vi "StimFile-Create.vi"(0 "File":T1, 7 "Npts":i32=-1, 11 "error in (no error)":errorcluster) -> (4 "File out":T1, 8 "Y":dbl[](array[numeric]), 15 "error out":errorcluster)   [LabVIEW 2020]
uses:
  StimFile-Params.ctl
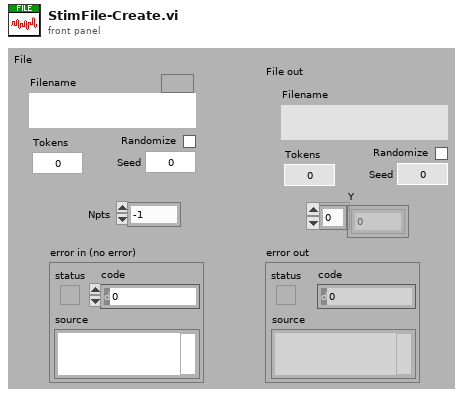
[diagram p1: front panel]
types:
  T1 = typedef "StimFile-Params.ctl" = cluster{"Filename":path, "Signal":dbl[], "Channel":i32, "stream":bool, "offset":i32, "nreps":i32, "loops":i32, "Randomize":bool, "order":i32[], "Seed":i32, "Tokens":i32}
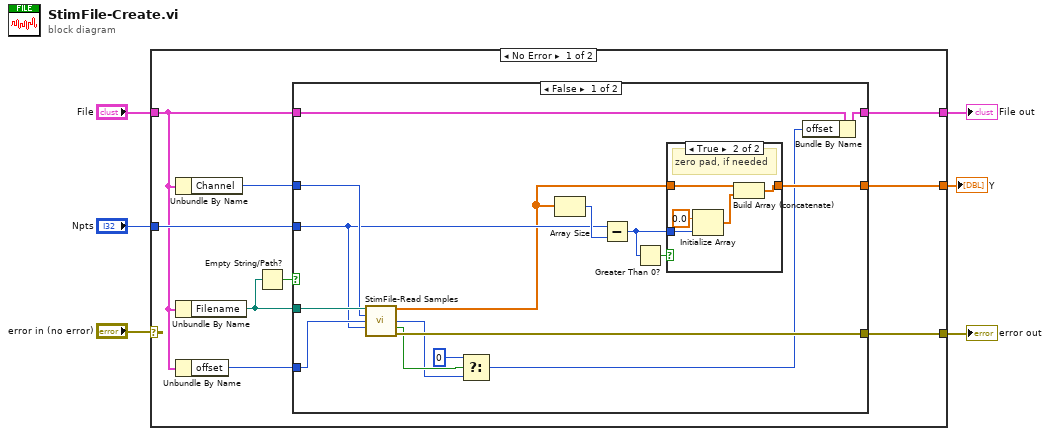
[diagram p0: block diagram]
diagram:
  n1 = case shown="No Error" "error in (no error)" {
    selector: "error in (no error)" -> [_ w39]
    tunnel: "File" -> [w9 _]
    tunnel: "Npts" -> [w14 _]
    tunnel: [w15 w39] -> w3
    tunnel: [w8 _] -> w2
    tunnel: [w7 _] -> w1
    frame No Error {
      n2 = Unbundle By Name(w9) -> ("Channel"=w11:i32)
      n3 = Unbundle By Name(w9) -> ("Filename"=w12:path)
      n4 = Unbundle By Name(w9) -> ("offset"=w10:i32)
      n5 = Empty String/Path?(string/path=w12) -> (empty?=w13:bool)
      n6 = case shown="False" w13 {
        tunnel: w12 -> [w31 _]
        tunnel: [w30 _] -> w15
        tunnel: w14 -> [w18 _]
        tunnel: w11 -> [w19 _]
        tunnel: w10 -> [w26 _]
        tunnel: w9 -> [w25 w38]
        tunnel: [w24 w38] -> w8
        tunnel: [w23 _] -> w7
        frame False {
          n7 = call "StimFile-Read Samples.vi"("Filename"=w31, "channel"=w19, "offset in"=w26, "Npts"=w18) -> ("Samples"=w16:dbl[], "offset out"=w17:i32, "end of file?"=w22:bool, "error out"=w30:errorcluster)  [unwired: 8 in]
          n8 = Select(t=0, s=w22, f=w17) -> (s? t:f=w21:i32)
          n9 = Array Size(array=w16) -> (size(s)=w29:i32)
          n10 = Subtract(x=w18, y=w29) -> (x-y=w27:i32)
          n11 = Greater Than 0?(x=w27) -> (x > 0?=w28:bool)
          n12 = case shown="True" w28 {
            tunnel: w16 -> [w32 w37]
            tunnel: w27 -> [_ w34]
            tunnel: [w32 w36] -> w23
            frame False {
            }
            frame True {
              # "zero pad, if needed"
              n13 = Initialize Array(0.0 ("element"), w34) -> (w35:dbl[])
              n14 = Build Array (concatenate)(w37, w35) -> (w36:dbl[])
            }
          }
          n15 = Bundle By Name(cluster=w25, "offset"=w21) -> (w24:T1)
        }
        frame True {
        }
      }
    }
    frame Error {
    }
  }
  "error out" <- w3
  "File out" <- w2
  "Y" <- w1
